vi "LoadImage.vi"(8 "error in (no error)":errorcluster, 10 "ImageData":T1, 11 "FaceRecognition in":refnum<class "FaceRecognition.lvclass">) -> (0 "error out":errorcluster, 2 "LoadImage":refnum<k24>, 3 "FaceRecognition out":refnum<class "FaceRecognition.lvclass">)   [LabVIEW 2020, in "FaceRecognitionDotNet.lvlib" / "FaceRecognition.lvclass"]
uses:
  FaceRecognition.lvclass
  ctl/ImageData.ctl
  dll/FaceRecognitionDotNet.dll
  FaceRecognition.lvclass/FaceRecognition.ctl
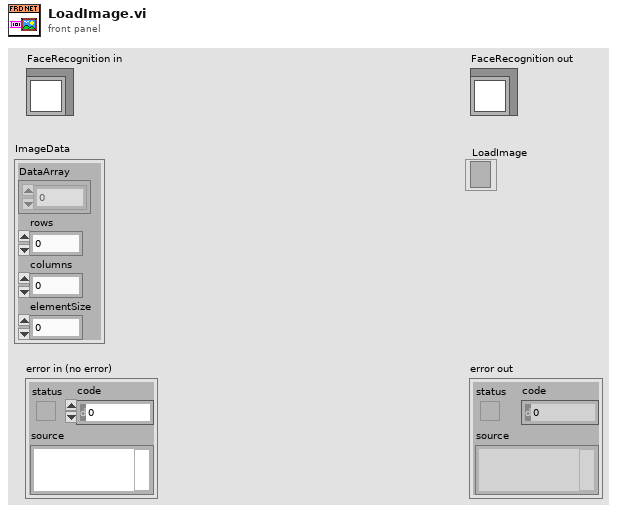
[diagram p1: front panel]
types:
  T1 = typedef "FaceRecognitionDotNet.lvlib/FaceRecognition.lvclass/ImageData.ctl" = cluster{"DataArray":u8[], "rows":i32, "columns":i32, "elementSize":i32}
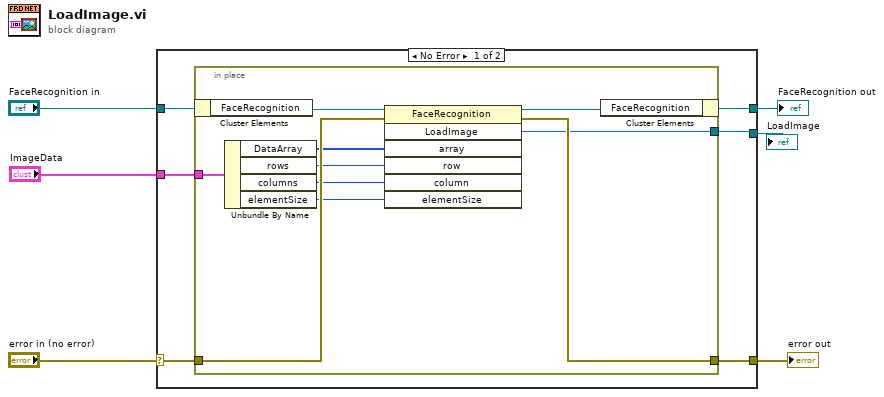
[diagram p0: block diagram]
diagram:
  n1 = case shown="No Error" "error in (no error)" {
    selector: "error in (no error)" -> [w10 w24]
    tunnel: [w9 w24] -> w5
    tunnel: [w11 w23] -> w3
    tunnel: "FaceRecognition in" -> [w12 w23]
    tunnel: [w8 _] -> w1
    tunnel: "ImageData" -> [w7 _]
    frame No Error {
      n2 = in-place {
        in-place-border: w10 -> [w20]
        in-place-border: [w19] -> w9
        in-place-border: [w18] -> w8
        in-place-border: w7 -> [w17]
        n3 = in-place-cluster #1(w12) -> ("FaceRecognition"=w22:refnum<k24>)
        n4 = Unbundle By Name(w17) -> ("DataArray"=w16:u8[], "rows"=w15:i32, "columns"=w14:i32, "elementSize"=w13:i32)
        n5 = invoke class="FaceRecognition" method="LoadImage"(reference=w22, error in=w20, "array"=w16, "row"=w15, "column"=w14, "elementSize"=w13) -> (reference out=w21:refnum<k24>, error out=w19:errorcluster, "LoadImage"=w18:refnum<k24>)  [unwired: 1 in, 4 out]
        n6 = in-place-cluster #1("FaceRecognition"=w21) -> (w11:refnum<class "FaceRecognition.lvclass">)
      }
    }
    frame Error {
    }
  }
  "error out" <- w5
  "FaceRecognition out" <- w3
  "LoadImage" <- w1
